vi "testDayRolloverEntriesGiveCorrectTotalDuration.vi"(8 "error in (no error)":errorcluster, 11 "TestCase in":refnum<class "FileLoadingTestCase.lvclass">) -> (0 "error out":errorcluster, 3 "TestCase out":refnum<class "FileLoadingTestCase.lvclass">)   [LabVIEW 2019, in "FileLoadingTestCase.lvclass"]
uses:
  FileLoadingTestCase.lvclass
  Sensors/Detector/Event.ctl
  <vilib>/Analysis/1siggen.llb/Ramp Pattern by Samples.vi
  <vilib>/addons/_JKI Toolkits/VI Tester/TestCase.llb/TestCase.lvclass
  Post-Processing/Muon Data Post-Processing.lvlib
  Logger/Logger/Logger.lvclass
  Sensors/Detector/Muon Detector.lvclass
  <vilib>/Analysis/NI_AALBase.lvlib
  C:/Program Files (x86)/National Instruments/LabVIEW 2019/vi.lib/addons/_JKI Toolkits/VI Tester/TestCase.llb/TestCase.lvclass
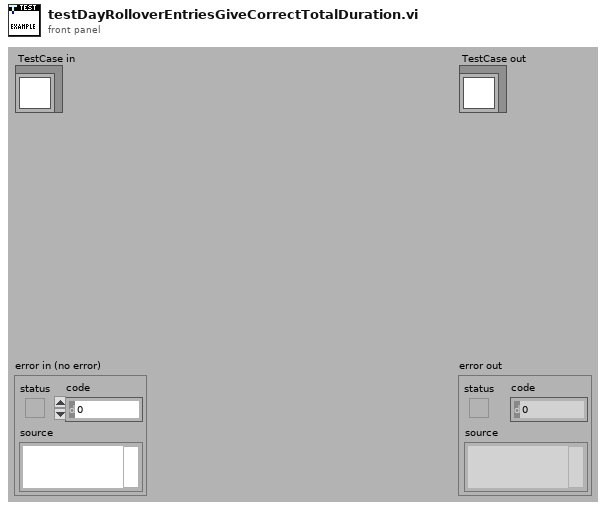
[diagram p1: front panel]
types:
  T1 = typedef "Muon Detector.lvclass/Event.ctl" = cluster{"Event Count":i32, "Device Timestamp (ms)":i32, "PC Timestamp":timestamp, "ADC Count":i32, "Event Type":u8}
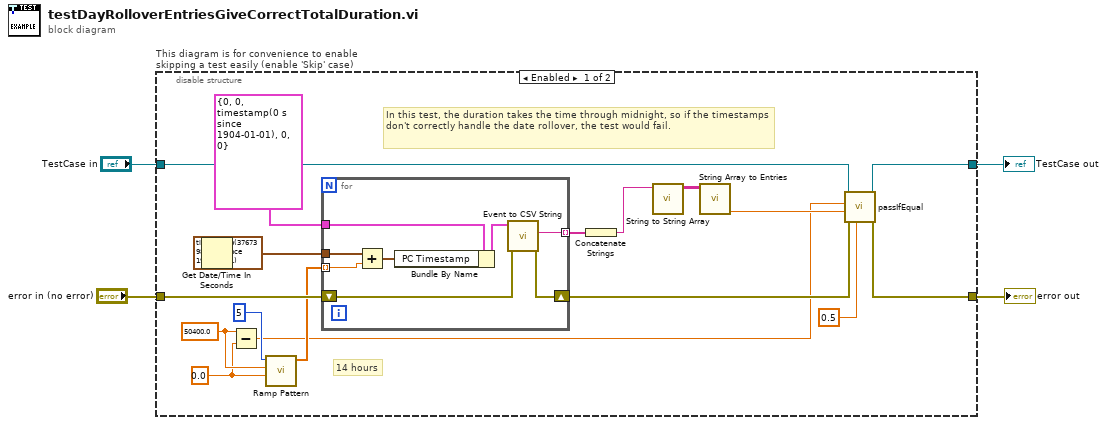
[diagram p0: block diagram]
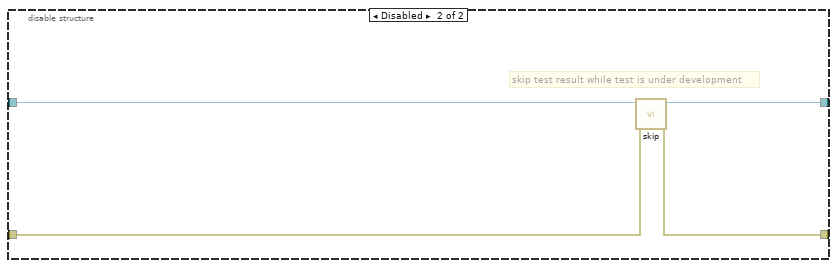
[diagram p2: hidden frame]
diagram:
  n1 = disable-structure "This diagram is for convenience to enable skipping a test easily (enable 'Skip' case)" shown="Enabled" {
    disable-tunnel: "TestCase in" -> [w21 w33]
    disable-tunnel: [w20 w31] -> w1
    disable-tunnel: [w19 w32] -> w3
    disable-tunnel: "error in (no error)" -> [w12 w30]
    frame Enabled {
      (unwired) timestamp(3767398200 s since 1904-01-01) ("current time")
      w7 = 50400.0 ("end")
      w6 = 0.0 ("start")
      # "14 hours"
      # "In this test, the duration takes the time through midnight, so if the timestamps don't correctly handle the date rollover, the test would fail."
      n2 = Get Date/Time In Seconds() -> (seconds since 1Jan1904=w8:timestamp)
      n3 = Subtract(x=w7, y=w6) -> (x-y=w5:dbl)
      n4 = call-poly <vilib>:"Ramp Pattern.vi"("start"=w6, "end"=w7, "samples"=5) -> ("Ramp Pattern"=w9:dbl[])  [unwired: 7 in, 1 out]
      n5 = for {
        tunnel: [w29] -> w15 mode=indexing
        shift-right: [w27] -> w13
        shift-left: w12 -> [w28]
        tunnel: T1 {"Event Count"=0, "Device Timestamp (ms)"=0, "PC Timestamp"=timestamp(0 s since 1904-01-01), "ADC Count"=0, "Event Type"=0} ("Event") -> [w26]
        tunnel: w9 -> [w24] mode=indexing
        tunnel: w8 -> [w22]
        n6 = Add(x=w22, y=w24) -> (x+y=w23:timestamp)
        n7 = Bundle By Name(cluster=w26, "PC Timestamp"=w23) -> (w25:T1)
        n8 = call "Event to CSV String.vi"("error in (no error)"=w28, "Event"=w25) -> ("error out"=w27:errorcluster, "String"=w29:string)  [unwired: 8 in]
      }
      n9 = Concatenate Strings(w15) -> (w14:string)
      n10 = call "String to String Array.vi"("String"=w14) -> ("Array"=w18:string[][])  [unwired: 10 in]
      n11 = call "String Array to Entries.vi"("String Array in"=w18) -> ("Total Duration"=w17:dbl)  [unwired: 7 in, 3 out]
      n12 = call-dynamic "passIfEqual.vi"("delta (optional)"=0.5, "error in (no error)"=w13, "y"=w17, "x"=w5, "TestCase in"=w21) -> ("error out"=w19:errorcluster, "TestCase out"=w20:refnum<class "FileLoadingTestCase.lvclass">)  [unwired: 5 in]
    }
    frame Disabled {
      # "skip test result while test is under development"
      n13 = call <vilib>:"skip.vi"("error in (no error)"=w30, "TestCase in"=w33) -> ("error out"=w32:errorcluster, "TestCase out"=w31:refnum<class "FileLoadingTestCase.lvclass">)  [unwired: 8 in]
    }
  }
  "error out" <- w3
  "TestCase out" <- w1
